vi "S2DS_Add single RC.vi"(6 "prefix in":string, 9 "RC Factor":dbl, 10 "RC instrument menu":string, 11 "RC name in":string) -> (1 "Prefix unit":string, 2 "Read channel info":T1, 4 "Base unit":string)   [LabVIEW 2025]
uses:
  TYPE DEFS/S2DS_Single RC info.ctl
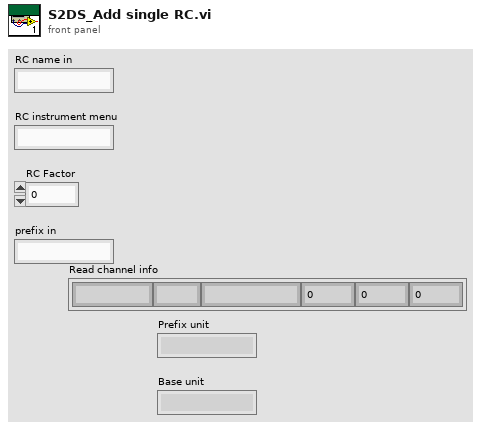
[diagram p1: front panel]
types:
  T1 = typedef "S2DS_Single RC info.ctl" = cluster{"Instrument identifier":string, "Factor":dbl, "Averaging":i32, "Wait (ms)":i32, "Unit":string, "Name":string}
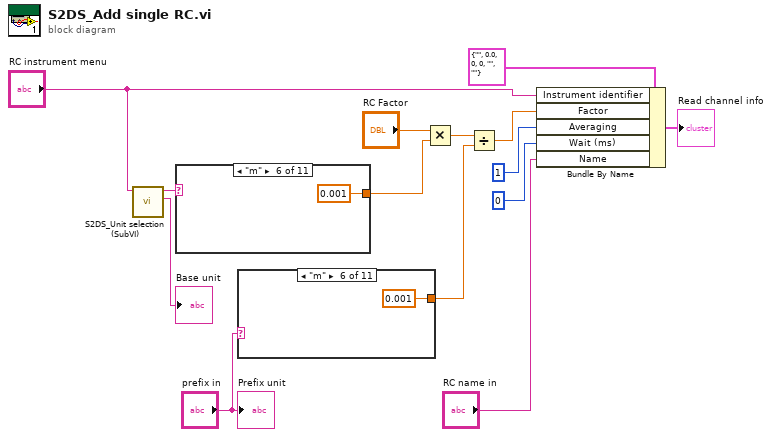
[diagram p0: block diagram]
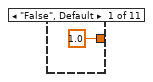
[diagram p2: hidden frame]
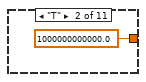
[diagram p3: hidden frame]
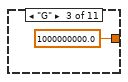
[diagram p4: hidden frame]
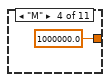
[diagram p5: hidden frame]
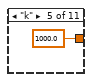
[diagram p6: hidden frame]
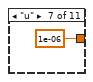
[diagram p7: hidden frame]
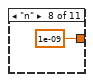
[diagram p8: hidden frame]
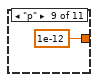
[diagram p9: hidden frame]
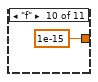
[diagram p10: hidden frame]
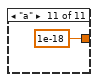
[diagram p11: hidden frame]
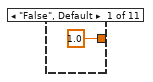
[diagram p12: hidden frame]
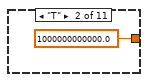
[diagram p13: hidden frame]
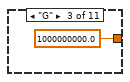
[diagram p14: hidden frame]
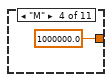
[diagram p15: hidden frame]
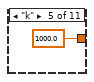
[diagram p16: hidden frame]
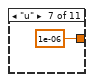
[diagram p17: hidden frame]
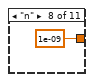
[diagram p18: hidden frame]
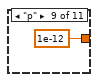
[diagram p19: hidden frame]
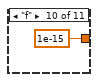
[diagram p20: hidden frame]
diagram:
  n1 = call "S2DS_Unit selection (SubVI).vi"("RC instrument name"="RC instrument menu") -> ("Base unit"=→"Base unit":string, "Instrument default prefix"=w8:string)  [unwired: 9 in]
  n2 = case shown="\"m\"" w8 {
    tunnel: [1.0 1000000000000.0 1000000000.0 1000000.0 1000.0 0.001 1e-06 1e-09 1e-12 1e-15 1e-18] -> w2
    frame "False", Default {
    }
    frame "T" {
    }
    frame "G" {
    }
    frame "M" {
    }
    frame "k" {
    }
    frame "m" {
    }
    frame "u" {
    }
    frame "n" {
    }
    frame "p" {
    }
    frame "f" {
    }
    frame "a" {
    }
  }
  n3 = case shown="\"m\"" "prefix in" {
    tunnel: [1.0 1000000000000.0 1000000000.0 1000000.0 1000.0 0.001 1e-06 1e-09 1e-12 1e-15 1e-18] -> w3
    frame "False", Default {
    }
    frame "T" {
    }
    frame "G" {
    }
    frame "M" {
    }
    frame "k" {
    }
    frame "m" {
    }
    frame "u" {
    }
    frame "n" {
    }
    frame "p" {
    }
    frame "f" {
    }
    frame "a" {
    }
  }
  n4 = Multiply(x="RC Factor", y=w2) -> (x*y=w1:dbl)
  n5 = Divide(x=w1, y=w3) -> (x/y=w9:dbl)
  n6 = Bundle By Name(cluster=T1 {"Instrument identifier"="", "Factor"=0.0, "Averaging"=0, "Wait (ms)"=0, "Unit"="", "Name"=""} ("Read channel info 2"), "Instrument identifier"="RC instrument menu", "Factor"=w9, "Averaging"=1, "Wait (ms)"=0, "Name"="RC name in") -> (→"Read channel info":T1)
  "Prefix unit" <- "prefix in"
